vi "ET3500 - Read Program.vi"(9 "subVI":bool=TRUE, 10 "Simulate":bool, 11 "VISA resource name":refnum<visa-resource-name>="visa://192.168.1.50/ASRL1::INSTR") -> (0 "error out":errorcluster, 2 "End(0) Segment#":i32=4, 3 "ET3500 Program":i32(listbox)=-1)   [LabVIEW 2013]
uses:
  Controls/ET3500 Enum.ctl
  Controls/ET3500 Programmer Enum.ctl
panel:
  in  "Graph":bool
  out "Status":string="Reading Successful."
  out "Slide":u8(slide)=133 scale=0.0..133.0
  in  "Stop Button":bool
  out "RampUnits":string="(secs)"
  out "DwellUnits":string="(min)"
  out "RampUnits":i16
  out "unscaled":i16[][](array[numeric])=[[1, 3, 1, 0, -32768, -32768, -32768, -32768, -32768, -32768, -32768, -32768, -32768, -32768, -32768, -32768], [-32768, 10, -32768, 0, -32768, -32768, -32768, -32768, -32768, -32768, -32768, -32768, -32768, -32768, -32768, -32768], [100, 0, 100, 0, -32768, -32768, -32768, -32768, -32768, -32768, -32768, -32768, -32768, -32768, -32768, -32768], [1, 1, 2, 0, -32768, -32768, -32768, -32768, -32768, -32768, -32768, -32768, -32768, -32768, -32768, -32768], [280, 50, 250, 5000, -32768, -32768, -32768, -32768, -32768, -32768, -32768, -32768, -32768, -32768, -32768, -32768], [-32768, -5536, -32768, 0, -32768, -32768, -32768, -32768, -32768, -32768, -32768, -32768, -32768, -32768, -32768, -32768], [1, 1, 2, 0, -32768, -32768, -32768, -32768, -32768, -32768, -32768, -32768, -32768, -32768, -32768, -32768], [280, 50, 250, 5000, -32768, -32768, -32768, -32768, -32768, -32768, -32768, -32768, -32768, -32768, -32768, -32768]]
  in  "ProgramNumber":i32=33
  out "VISA resource name out":refnum<visa-resource-name>="visa://192.168.1.50/ASRL1::INSTR"
  out "DwellUnits":i16=1
  out "ET3504 Program Number":i16=33
  out "ProgramNumber":i16=33
  out "ProgStatus":i16=1
  # "Duration, RampRate/hour,\n TargetSP,GSoakVal\nall x10"
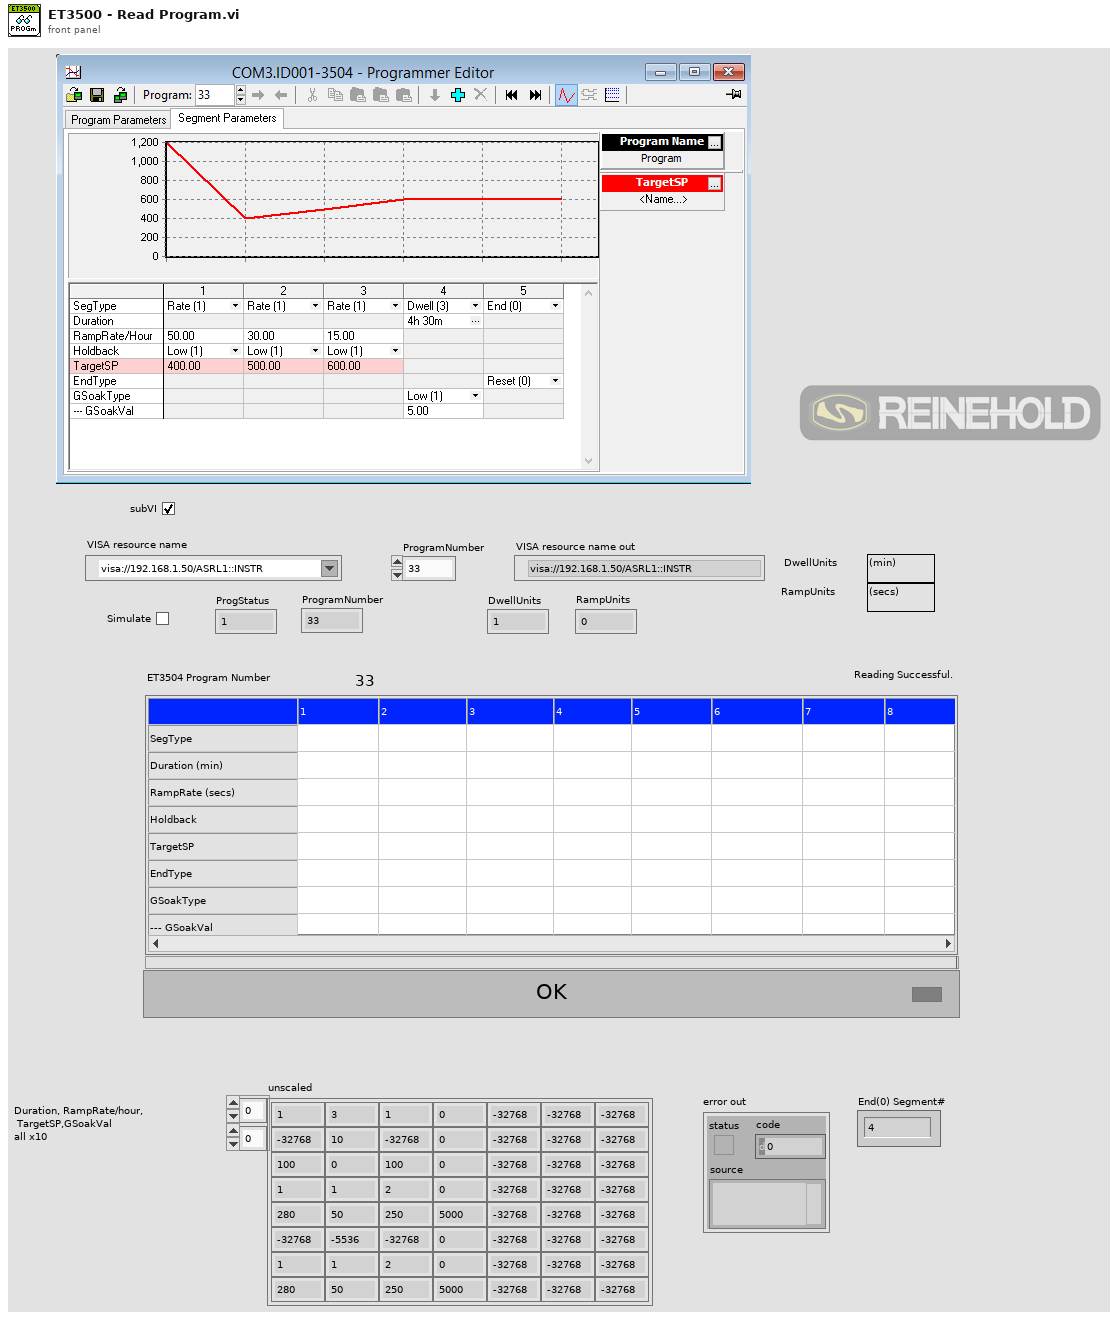
[diagram p1: front panel]
types:
  T1 = typedef "ET3500 Programmer Enum.ctl" = u16
  T2 = typedef "ET3500 Enum.ctl" = enum16{"Programmer1", "Segment1", "Segment2", "Segment3", "Segment4", "Segment5", "Segment6", "Segment7", "Segment8", "Segment9", "Segment10", "Segment11", "Segment12", "Segment13", "Segment14", "Segment15", "Segment16"}
  T3 = enum8{"Enabled", "Disabled", "Disabled and Grayed Out"}
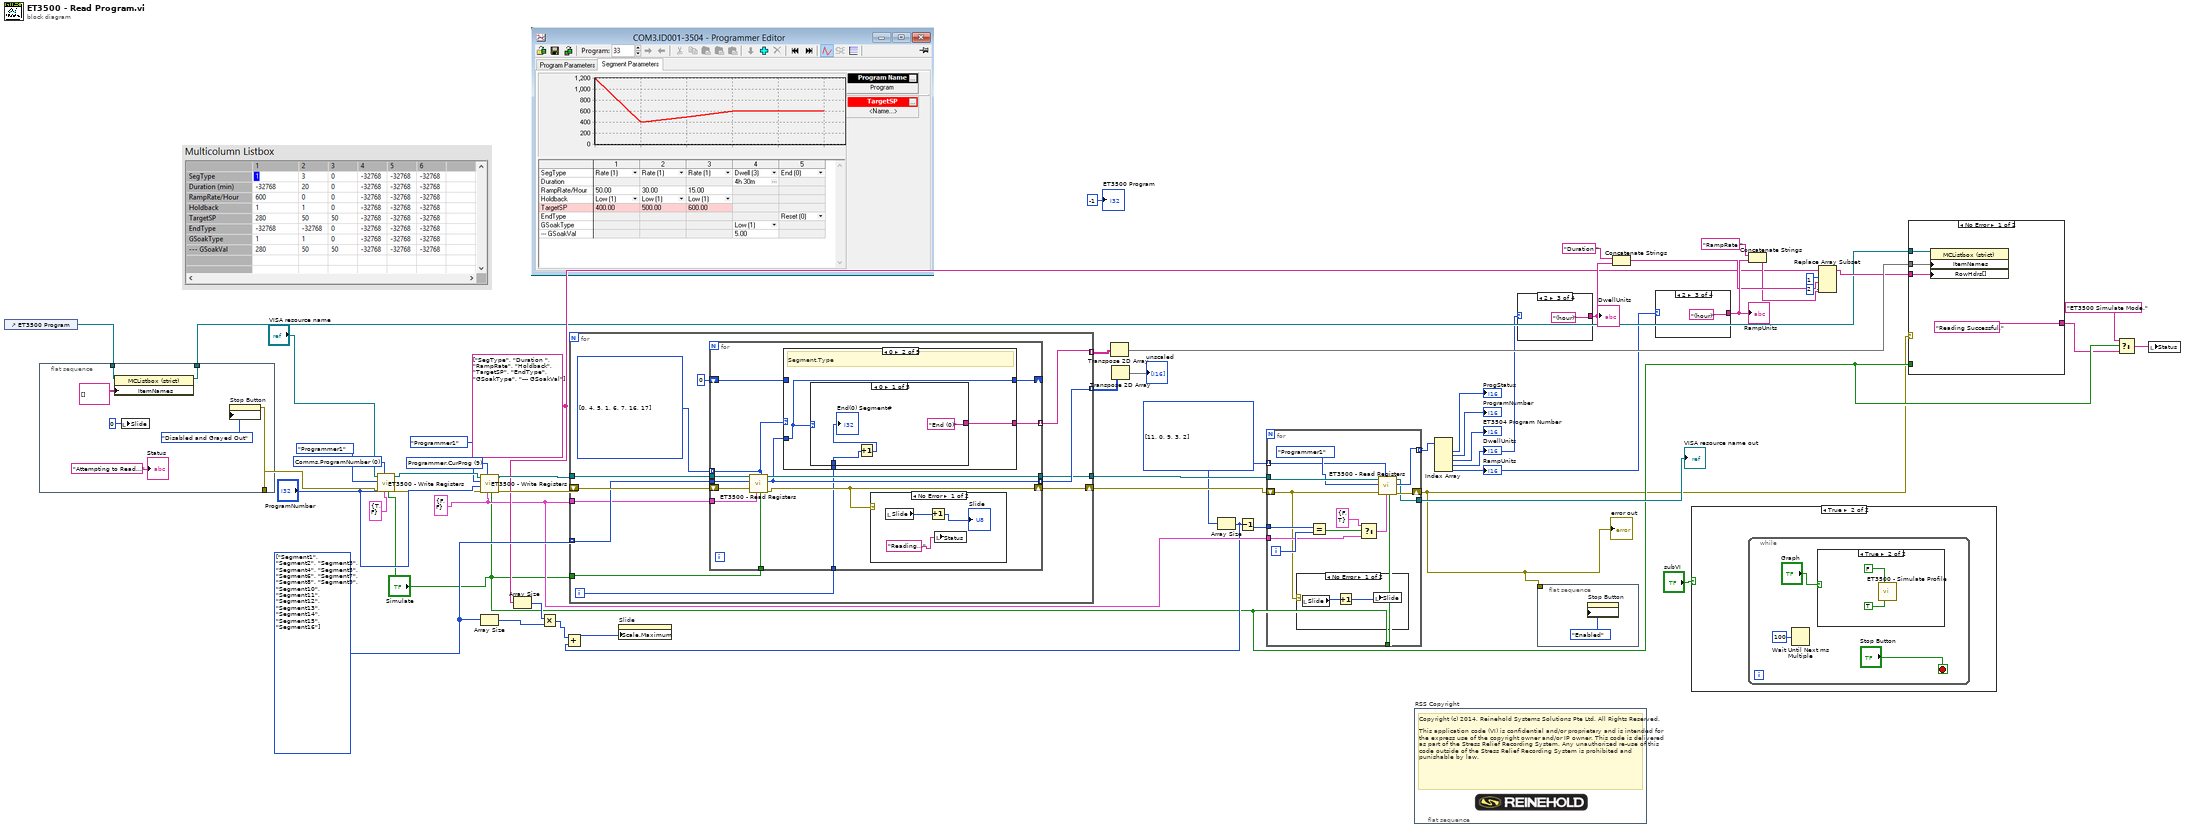
[diagram p0: block diagram]
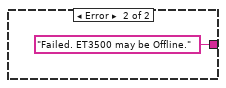
[diagram p3: hidden frame]
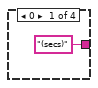
[diagram p6: hidden frame]
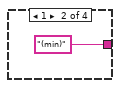
[diagram p7: hidden frame]
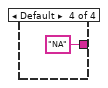
[diagram p8: hidden frame]
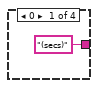
[diagram p9: hidden frame]
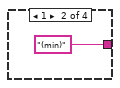
[diagram p10: hidden frame]
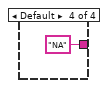
[diagram p11: hidden frame]
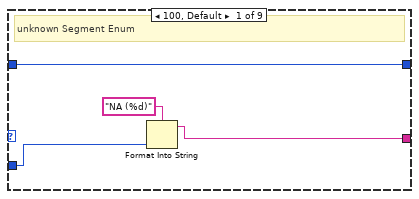
[diagram p13: hidden frame]
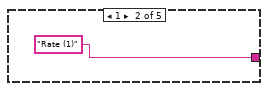
[diagram p14: hidden frame]
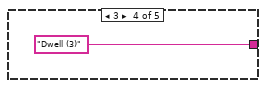
[diagram p16: hidden frame]
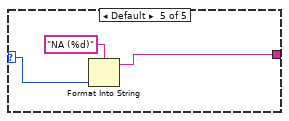
[diagram p17: hidden frame]
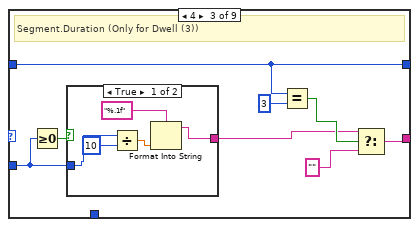
[diagram p18: hidden frame]
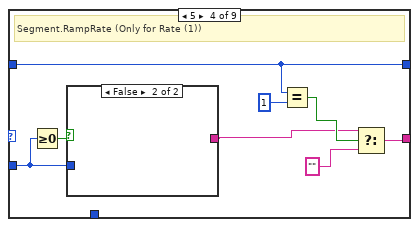
[diagram p20: hidden frame]
diagram:
  w16 = T1[] [11, 0, 9, 3, 2] items=["Comms.ProgramNumber", "", "Program.RampUnits", "Program.DwellUnits", "", "", "", "", "", "Programmer.CurProg", "Programmer.CurSeg", "Programmer.ProgStatus", "", "", "", "", "", "Programmer.ProgTimeLeft", "Programmer.PVIn", "Programmer.SPIn", "", "Programmer.SegTimeLeft"]
  w27 = string[] ["SegType", "Duration ", "RampRate", "Holdback", "TargetSP", "EndType", "GSoakType", "--- GSoakVal"] ("Row Header Strings[]")
  w14 = cluster{"Init":bool, "Close":bool} {"Init"=FALSE, "Close"=FALSE} ("Option")
  w51 = T1 0 items=["Comms.ProgramNumber", "", "Program.RampUnits", "Program.DwellUnits", "", "", "", "", "", "Programmer.CurProg", "Programmer.CurSeg", "Programmer.ProgStatus", "", "", "", "", "", "Programmer.ProgTimeLeft", "Programmer.PVIn", "Programmer.SPIn", "", "Programmer.SegTimeLeft"] ("ET3500 Programmer Enum")
  w45 = T1 9 items=["Comms.ProgramNumber", "", "Program.RampUnits", "Program.DwellUnits", "", "", "", "", "", "Programmer.CurProg", "Programmer.CurSeg", "Programmer.ProgStatus", "", "", "", "", "", "Programmer.ProgTimeLeft", "Programmer.PVIn", "Programmer.SPIn", "", "Programmer.SegTimeLeft"] ("ET3500 Programmer Enum")
  w28 = T2[] [enum."Segment1", enum."Segment2", enum."Segment3", enum."Segment4", enum."Segment5", enum."Segment6", enum."Segment7", enum."Segment8", enum."Segment9", enum."Segment10", enum."Segment11", enum."Segment12", enum."Segment13", enum."Segment14", enum."Segment15", enum."Segment16"] items=["Programmer1", "Segment1", "Segment2", "Segment3", "Segment4", "Segment5", "Segment6", "Segment7", "Segment8", "Segment9", "Segment10", "Segment11", "Segment12", "Segment13", "Segment14", "Segment15", "Segment16"]
  n1 = control-ref of="ET3500 Program"() -> (w22:refnum<vi>)
  n2 = flat-sequence {
    tunnel: [w59] -> w23
    tunnel: w22 -> [w58]
    tunnel: [w57] -> w21
    frame #0 {
      n3 = property class="MCListbox (strict)"(reference=w58, "ItemNames"=string[][] [] ("Item Names")) -> (reference out=w57:refnum<vi>)  [unwired: 1 in, 1 out]
      n4 = local write "Slide"(u8 0 ("Slide")) -> ()
      n5 = property on="Stop Button" class="Bool"("DisabledEnum"=T3."Disabled and Grayed Out" ("Disabled")) -> (error out=w59:errorcluster)  [unwired: 2 in, 1 out]
      "Status" <- "Attempting to Read..." ("Status")
    }
  }
  n6 = call "ET3500 - Write Registers.vi"("Simulate"="Simulate", "Option"=cluster{"Init":bool, "Close":bool} {"Init"=TRUE, "Close"=FALSE}, "ET3500 Programmer Enum"=w51, "error in (no error)"=w23, "Process Variable  (0)"="ProgramNumber", "ET3500 Enum"=ET3500_Enum."Programmer1", "VISA resource name"="VISA resource name") -> ("error out"=w20:errorcluster, "VISA resource name out"=w49:refnum<visa-resource-name>)  [unwired: 3 in]
  n7 = call "ET3500 - Write Registers.vi"("Simulate"="Simulate", "Option"=w14, "ET3500 Programmer Enum"=w45, "error in (no error)"=w20, "Process Variable  (0)"="ProgramNumber", "ET3500 Enum"=ET3500_Enum."Programmer1", "VISA resource name"=w49) -> ("error out"=w47:errorcluster, "VISA resource name out"=w50:refnum<visa-resource-name>)  [unwired: 3 in]
  n8 = Array Size(array=w28) -> (size(s)=w26:i32)
  n9 = Array Size(array=w27) -> (size(s)=w25:i32)
  n10 = Multiply(x=w25, y=w26) -> (x*y=w24:i32)
  n11 = for {
    tunnel: w28 -> [w70] mode=indexing
    tunnel: w50 -> [w72]
    shift-right: [w69] -> w18
    shift-left: w47 -> [w71]
    tunnel: "Simulate" -> [w66]
    tunnel: [w68] -> w53 mode=indexing
    tunnel: [w67] -> w17
    tunnel: w14 -> [w65]
    tunnel: [w63] -> w42 mode=indexing
    i -> [w61]
    w64 = u16[] [0, 4, 5, 1, 6, 7, 16, 17] items=["Segment.Type", "Segment.Holdback", "", "", "Segment.Duration", "Segment.RampRate", "Segment.TargetSP", "Segment.EndAction", "", "", "", "", "", "", "", "", "Segment.GsoakType", "Segment.GsoakVal"]
    n12 = for {
      tunnel: w72 -> [w85]
      tunnel: w66 -> [w83]
      tunnel: w70 -> [w74]
      tunnel: w65 -> [w82]
      tunnel: w64 -> [w80] mode=indexing
      tunnel: [w79] -> w68 mode=indexing
      shift-right: [w77] -> w69
      shift-left: w71 -> [w84]
      tunnel: [w81] -> w67
      tunnel: [w78] -> w63 mode=indexing
      shift-right: [w76] -> _
      shift-left: i16 0 ("Data") -> [w75]
      tunnel: w61 -> [w73]
      n13 = call "ET3500 - Read Registers.vi"("Simulate"=w83, "ET3500 Segment Enum"=w80, "Option"=w82, "error in (no error)"=w84, "ET3500 Enum"=w74, "VISA resource name"=w85) -> ("error out"=w77:errorcluster, "Data"=w79:i16, "VISA resource name out"=w81:refnum<visa-resource-name>)  [unwired: 2 in, 1 out]
      n14 = case shown="0" w80 {
        tunnel: w79 -> [w91 w94 w110 w123 w136 w148 w161 w172 w183]
        tunnel: [w90 w95 w104 w118 w130 w143 w156 w167 w178] -> w78
        tunnel: [w89 w94 w109 w117 w132 w142 w155 w166 w177] -> w76
        tunnel: w75 -> [w89 _ w109 w117 w132 w142 w155 w166 w177]
        tunnel: w73 -> [_ w93 _ _ _ _ _ _ _]
        frame 100, Default {
          # "unknown Segment Enum"
          n15 = Format Into String(format string="NA (%d)", w91) -> (resulting string=w90:string)  [unwired: 2 in, 1 out]
        }
        frame 0 {
          # "Segment.Type"
          n16 = case shown="0" w94 {
            selector: w94 -> [_ _ _ _ w102]
            tunnel: ["End (0)" "Rate (1)" _ "Dwell (3)" w101] -> w95
            tunnel: w93 -> [w97 _ _ _ _]
            frame 0 {
              n17 = Increment(x=w97) -> (x+1=→"End(0) Segment#":i32)
            }
            frame 1 {
            }
            frame ..-1 {
            }
            frame 3 {
            }
            frame Default {
              n18 = Format Into String(format string="NA (%d)", w102) -> (resulting string=w101:string)  [unwired: 2 in, 1 out]
            }
          }
        }
        frame 4 {
          # "Segment.Duration (Only for Dwell (3))"
          n19 = Greater Or Equal To 0?(x=w110) -> (x >= 0?=w111:bool)
          n20 = case shown="True" w111 {
            tunnel: [w112 _] -> w106
            tunnel: w110 -> [w116 _]
            frame True {
              n21 = Divide(x=w116, y=i16 10) -> (x/y=w114:dbl)
              n22 = Format Into String(format string="%.1f", w114) -> (resulting string=w112:string)  [unwired: 2 in, 1 out]
            }
            frame False {
            }
          }
          n23 = Equal?(x=w109, y=i16 3) -> (x = y?=w107:bool)
          n24 = Select(t=w106, s=w107, f="") -> (s? t:f=w104:string)
        }
        frame 5 {
          # "Segment.RampRate (Only for Rate (1))"
          n25 = Greater Or Equal To 0?(x=w123) -> (x >= 0?=w124:bool)
          n26 = case shown="False" w124 {
            tunnel: [w125 _] -> w119
            tunnel: w123 -> [w129 _]
            frame True {
              n27 = Divide(x=w129, y=i16 10) -> (x/y=w127:dbl)
              n28 = Format Into String(format string="%.1f ", w127) -> (resulting string=w125:string)  [unwired: 2 in, 1 out]
            }
            frame False {
            }
          }
          n29 = Equal?(x=w117, y=i16 1) -> (x = y?=w121:bool)
          n30 = Select(t=w119, s=w121, f="") -> (s? t:f=w118:string)
        }
        frame 1 {
          # "Segment.Holdback (Only for Rate (1))"
          n31 = case shown="Default" w136 {
            selector: w136 -> [_ _ _ w140]
            tunnel: [_ "Low (1)" "High (2)" w139] -> w131
            frame ..-1 {
            }
            frame 1 {
            }
            frame 2 {
            }
            frame Default {
              n32 = Format Into String(format string="NA (%d)", w140) -> (resulting string=w139:string)  [unwired: 2 in, 1 out]
            }
          }
          n33 = Equal?(x=w132, y=i16 1) -> (x = y?=w134:bool)
          n34 = Select(t=w131, s=w134, f="") -> (s? t:f=w130:string)
        }
        frame 6 {
          # "TargetSP (Only for Rate (1))"
          n35 = Greater Or Equal To 0?(x=w148) -> (x >= 0?=w149:bool)
          n36 = case shown="True" w149 {
            tunnel: [w150 _] -> w144
            tunnel: w148 -> [w154 _]
            frame True {
              n37 = Divide(x=w154, y=i16 10) -> (x/y=w152:dbl)
              n38 = Format Into String(format string="%.1f ", w152) -> (resulting string=w150:string)  [unwired: 2 in, 1 out]
            }
            frame False {
            }
          }
          n39 = Equal?(x=w142, y=i16 1) -> (x = y?=w146:bool)
          n40 = Select(t=w144, s=w146, f="") -> (s? t:f=w143:string)
        }
        frame 7 {
          # "Segment.EndAction (EndType) (Only for End(0))"
          n41 = case shown="Default" w161 {
            selector: w161 -> [_ _ w164]
            tunnel: [_ "Reset (0)" w163] -> w157
            frame ..-1 {
            }
            frame 0 {
            }
            frame Default {
              n42 = Format Into String(format string="NA (%d)", w164) -> (resulting string=w163:string)  [unwired: 2 in, 1 out]
            }
          }
          n43 = Equal?(x=w155, y=i16 0) -> (x = y?=w159:bool)
          n44 = Select(t=w157, s=w159, f="") -> (s? t:f=w156:string)
        }
        frame 16 {
          # "Segment.GsoakType (Ony for Dwell (3))"
          n45 = case shown="Default" w172 {
            selector: w172 -> [_ _ w175]
            tunnel: [_ "Low (1)" w174] -> w168
            frame ..-1 {
            }
            frame 1 {
            }
            frame Default {
              n46 = Format Into String(format string="NA (%d)", w175) -> (resulting string=w174:string)  [unwired: 2 in, 1 out]
            }
          }
          n47 = Equal?(x=w166, y=i16 3) -> (x = y?=w170:bool)
          n48 = Select(t=w168, s=w170, f="") -> (s? t:f=w167:string)
        }
        frame 17 {
          # "--- GSoakVal (Only for Dwell (3))"
          n49 = case shown="Default" w183 {
            selector: w183 -> [w184 _]
            tunnel: [w185 _] -> w179
            frame Default {
              n50 = Divide(x=w184, y=i16 10) -> (x/y=w187:dbl)
              n51 = Format Into String(format string="%.1f ", w187) -> (resulting string=w185:string)  [unwired: 2 in, 1 out]
            }
            frame ..-1 {
            }
          }
          n52 = Equal?(x=w177, y=i16 3) -> (x = y?=w181:bool)
          n53 = Select(t=w179, s=w181, f="") -> (s? t:f=w178:string)
        }
      }
      n54 = case shown="No Error" w77 {
        frame No Error {
          n55 = local read "Slide"() -> (w87:u8)
          n56 = Increment(x=w87) -> (x+1=→"Slide":u8)
          n57 = local write "Status"("Reading..." ("Status")) -> ()
        }
        frame Error {
        }
      }
    }
  }
  n58 = Transpose 2D Array(2D array=w42) -> (transposed array=w39:string[][])
  n59 = Transpose 2D Array(2D array=w53) -> (transposed array=→"unscaled":i16[][])
  n60 = Array Size(array=w16) -> (size(s)=w6:i32)
  n61 = Add(x=w24, y=w6) -> (x+y=w19:i32)
  n62 = property on="Slide" class="Slide (strict)"("Scale.Maximum"=w19) -> ()  [unwired: 2 in, 2 out]
  n63 = Decrement(x=w6) -> (x-1=w15:i32)
  n64 = for {
    tunnel: w16 -> [w199] mode=indexing
    shift-right: [w202] -> w1
    shift-left: w18 -> [w189]
    tunnel: w17 -> [w201]
    tunnel: [w198] -> w13 mode=indexing
    tunnel: w15 -> [w197]
    tunnel: w14 -> [w193]
    tunnel: "Simulate" -> [w191]
    tunnel: [w190] -> w8
    i -> [w196]
    n65 = case shown="No Error" w189 {
      frame No Error {
        n66 = local read "Slide"() -> (w204:u8)
        n67 = Increment(x=w204) -> (x+1=w203:u8)
        n68 = local write "Slide"(w203) -> ()
      }
      frame Error {
      }
    }
    n69 = Equal?(x=w197, y=w196) -> (x = y?=w195:bool)
    n70 = Select(t=cluster{"Init":bool, "Close":bool} {"Init"=FALSE, "Close"=TRUE} ("Option"), s=w195, f=w193) -> (s? t:f=w192:cluster{"Init":bool, "Close":bool})
    n71 = call "ET3500 - Read Registers.vi"("Simulate"=w191, "Option"=w192, "ET3500 Programmer Enum"=w199, "error in (no error)"=w189, "ET3500 Enum"=ET3500_Enum."Programmer1", "VISA resource name"=w201) -> ("error out"=w202:errorcluster, "Data"=w198:i16, "VISA resource name out"=w190:refnum<visa-resource-name>)  [unwired: 2 in, 1 out]
  }
  "error out" <- w1
  "VISA resource name out" <- w8
  n72 = flat-sequence "RSS Copyright" {
    frame #0 {
      # "Copyright (c) 2014, Reinehold Systems Solutions Pte Ltd. All Rights Reserved.\n\nThis application code (VI) is confidential and/or proprietary and is intended for the express use of the copyright owner and/or IP owner. This code is delivered as part of the Stress Relief Recording System. Any unauthorized re-use of this code outside of the Stress Relief Recording System is prohibited and punishable by law."
    }
  }
  n73 = Index Array(array=w13) -> (element #1=→"ProgStatus":i16, element #2=→"ProgramNumber":i16, element #3=→"ET3504 Program Number":i16, element #4=w7:i16, element #5=w9:i16)  [unwired: 5 in]
  "DwellUnits" <- w7
  "RampUnits" <- w9
  n74 = case shown="2" w7 {
    tunnel: ["(secs)" "(min)" "(hour)" "NA"] -> w35
    frame 0 {
    }
    frame 1 {
    }
    frame 2 {
    }
    frame Default {
    }
  }
  "DwellUnits" <- w35
  n75 = flat-sequence {
    tunnel: w1 -> [_]
    frame #0 {
      n76 = property on="Stop Button" class="Bool"("DisabledEnum"=T3."Enabled" ("Disabled")) -> ()  [unwired: 2 in, 2 out]
    }
  }
  n77 = Concatenate Strings("Duration " ("String"), w35) -> (w32:string)
  n78 = case shown="2" w9 {
    tunnel: ["(secs)" "(min)" "(hour)" "NA"] -> w33
    frame 0 {
    }
    frame 1 {
    }
    frame 2 {
    }
    frame Default {
    }
  }
  "RampUnits" <- w33
  n79 = case shown="True" "subVI" {
    frame False {
    }
    frame True {
      n80 = while {
        stop <- "Stop Button" stop-if-true
        n81 = Wait Until Next ms Multiple(millisecond multiple=u32 100) -> ()  [unwired: 1 out]
        n82 = case shown="True" "Graph" {
          frame False {
          }
          frame True {
            n83 = call "ET3500 - Simulate Profile.vi"("Popup"=TRUE ("subVI"), "Set (T) / Get (F)"=FALSE) -> ()  [unwired: 5 in, 5 out]
          }
        }
      }
    }
  }
  n84 = Concatenate Strings("RampRate " ("String"), w33) -> (w30:string)
  n85 = Replace Array Subset(array=w27, new element #1=w32, index #1=1 ("index"), new element #2=w30, index #2=2 ("index")) -> (w29:string[])
  n86 = case shown="No Error" w1 {
    tunnel: w39 -> [w222 _]
    tunnel: w29 -> [w221 _]
    tunnel: w21 -> [w220 _]
    tunnel: ["Reading Successful." ("Status") "Failed. ET3500 may be Offline." ("Status")] -> w4
    tunnel: "Simulate" -> [_ _]
    frame No Error {
      n87 = property class="MCListbox (strict)"(reference=w220, "ItemNames"=w222, "RowHdrs[]"=w221) -> ()  [unwired: 1 in, 2 out]
    }
    frame Error {
    }
  }
  n88 = Select(t="ET3500 Simulate Mode.", s="Simulate", f=w4) -> (s? t:f=w3:string)
  n89 = local write "Status"(w3) -> ()
  "ET3500 Program" <- -1 ("ET3500 Program")
